vi "Main_ver4.vi"(0 "PID On":bool) -> (5 "Total (V)":dbl[](array[slide]) scale=-8.0..8.0, 6 "Force (N)":T1(graph)={"M1 ref force"=19.748953974895397, "M2 ref force"=19.748953974895397, "M1 mes force"=8.73009296352717, "M2 mes force"=8.373055442726807})   [LabVIEW 2021]
uses:
  <vilib>/addons/control/pid/NI_PID_pid.lvlib
  <vilib>/platform/TimedLoop/XDataNode/XDataNode.xnode
  <vilib>/Platform/TimedLoop/XDataNode/nitl_modes.ctl
  <vilib>/Platform/TimedLoop/XDataNode/XDNodeRunTimeDep.lvlib
  <vilib>/Platform/TimedLoop/XDataNode/wakeup.ctl
  <vilib>/Platform/TimedLoop/XDataNode/timing_clust.ctl
  <vilib>/Analysis/NI_AALBase.lvlib
  <vilib>/DAQmx/configure/timing.llb/DAQmx Timing (Sample Clock).vi
  <vilib>/ptbypt/NI_PtbyPt.lvlib
  <vilib>/Analysis/3filter.llb/Filter Passband Type.ctl
  <vilib>/DAQmx/create/channels.llb/DAQmx Create Channel (AI-Voltage-Basic).vi
  <vilib>/DAQmx/create/channels.llb/DAQmx Create Channel (DO-Digital Output).vi
  <vilib>/addons/control/pid/pid.llb/PID (DBL).vi
  <vilib>/DAQmx/write.llb/DAQmx Write (Digital 1D Bool 1Chan 1Samp).vi
  <vilib>/Analysis/baseanly.llb/Real Dot Product.vi
  <vilib>/DAQmx/write.llb/DAQmx Write (Analog 1D DBL NChan 1Samp).vi
  <vilib>/DAQmx/create/channels.llb/DAQmx Create Channel (AO-Voltage-Basic).vi
panel:
  in  "Tab":enum32{"Page 1", "Page 2"}(tab)
  out "RBF Output":dbl(slide)=-2.8000715957430593 scale=-40.0..50.0
  out "Speed":dbl[](array[numeric])=[1.7549382010467513e-60, 1.807415273169756e-52]
  out "Mes Tension":dbl[](array[numeric])=[10.779007592916166, 8.389554321602144]
  out "Mes Position (mm)":dbl[](array[numeric])=[75.36000199819, -48.33317799163001]
  out "Ref Position (mm)":dbl
  out "Ref Tension":dbl[](array[numeric])=[19.748953974895397, 19.748953974895397]
  in  "Tab Control 4":enum32{"GRAPH", "DEVEL"}(tab)
  out "XY Graph":cluster{dbl[], dbl[]}[](graph)=[{[0.0, 26.31578947368421, 52.63157894736842, 78.94736842105263, 105.26315789473684, 131.57894736842104, 157.89473684210526, 184.21052631578945, 210.52631578947367, 236.8421052631579, 263.1578947368421, 289.4736842105263, 315.7894736842105, 342.10526315789474, 368.4210526315789, 394.7368421052631, 421.05263157894734, 447.36842105263156, 473.6842105263158, 499.99999999999994], [-1.87, -1.8414422208867078, -1.7583590718201578, -1.6281335147614857, -1.4618588659589593, -1.2727815045556152, -1.0745713204427367, -0.879730430835235, -0.6983883150844216, -0.5376223240442685, -0.40131981493157487, -0.2904938166741144, -0.20389950050143207, -0.13878048824938563, -0.09159539506910583, -0.058620814615532306, -0.03638002877625406, -0.02189309729851222, -0.012775689731560116, -0.007229270660814157]}, {[0.0, 26.31578947368421, 52.63157894736842, 78.94736842105263, 105.26315789473684, 131.57894736842104, 157.89473684210526, 184.21052631578945, 210.52631578947367, 236.8421052631579, 263.1578947368421, 289.4736842105263, 315.7894736842105, 342.10526315789474, 368.4210526315789, 394.7368421052631, 421.05263157894734, 447.36842105263156, 473.6842105263158, 499.99999999999994], [-0.5809906464511002, -0.7664296918795039, -0.9804116917090333, -1.2161233359855126, -1.462782454638376, -1.706140698730468, -1.9296694582665639, -2.116332899482121, -2.2507021378374863, -2.3210529255377237, -2.3210529255377237, -2.2507021378374863, -2.1163328994821216, -1.9296694582665639, -1.7061406987304686, -1.4627824546383765, -1.2161233359855128, -0.9804116917090334, -0.7664296918795039, -0.5809906464511005]}, {[0.0, 26.31578947368421, 52.63157894736842, 78.94736842105263, 105.26315789473684, 131.57894736842104, 157.89473684210526, 184.21052631578945, 210.52631578947367, 236.8421052631579, 263.1578947368421, 289.4736842105263, 315.7894736842105, 342.10526315789474, 368.4210526315789, 394.7368421052631, 421.05263157894734, 447.36842105263156, 473.6842105263158, 499.99999999999994], [0.006649382639893229, 0.011750901785178288, 0.020136966499166315, 0.03346184464981654, 0.05391861023460723, 0.08424817086570154, 0.12764836352349906, 0.18754392559490007, 0.2671921736253885, 0.3691283859263683, 0.49449753869312374, 0.6423678620027834, 0.8091638187361518, 0.9883757599794155, 1.1706867314629184, 1.3445974595986148, 1.4975345697271418, 1.6173142264869897, 1.6937329518316242, 1.72]}, {[0.0, 26.31578947368421, 52.63157894736842, 78.94736842105263, 105.26315789473684, 131.57894736842104, 157.89473684210526, 184.21052631578945, 210.52631578947367, 236.8421052631579, 263.1578947368421, 289.4736842105263, 315.7894736842105, 342.10526315789474, 368.4210526315789, 394.7368421052631, 421.05263157894734, 447.36842105263156, 473.6842105263158, 499.99999999999994], [-2.444341263811207, -2.5961210109810335, -2.7186337970300247, -2.8107950060971816, -2.8707227103627284, -2.8946740324203812, -2.8765924151858018, -2.808519404722456, -2.6818982792965196, -2.489546863655624, -2.2278752017761745, -1.898828092508817, -1.5110685812474018, -1.080074186536534, -0.627049362336656, -0.17680580965529402, 0.2450312049653749, 0.6150094374794441, 0.9145275702205602, 1.1317800828880853]}]
  in  "RBF":cluster{"STD":dbl, "Number":i32}={"STD"=150.0, "Number"=3}
  out "Weights":dbl[](array[slide])=[-1.87, -2.33, 1.72] scale=0.0..100.0
  in  "State x":cluster{"Number":i32, "x_0":dbl, "x_f":dbl}={"Number"=20, "x_0"=0.0, "x_f"=500.0}
  in  "Initialize":bool
  in  "Init Loadcell":bool
  out "Period":i64=2
  out "Finished Late? [i-1]":bool
  in  "Set Tension":dbl
  in  "Record?":bool
  in  "Trajectory":i32(knob) scale=0.0..2.0
  in  "Tab Control":enum32{"FORCE", "EE POS", "SPEED"}(tab)=enum."EE POS"
  out "Position (mm)":cluster{"Position":dbl, "Output (mm)":dbl}(graph)={"Position"=75.36000199819, "Output (mm)"=0.0}
  out "RPM":cluster{"Filtered x":dbl, "Filtered x":dbl}(graph)={"Filtered x"=1.7549382010467513e-60, "Filtered x"=1.807415273169756e-52}
  in  "RBF":bool=TRUE
  in  "Set Point":dbl(slide)=19.748953974895397 scale=0.0..40.0
  in  "stop":bool
  in  "Tab Control 3":enum32{"SPEED", "ENABLE", "POSITION"}(tab)
  in  "Gains":T2(array[cluster])=[{"proportional gain (Kc)"=0.03, "integral time (Ti, min)"=0.0, "derivative time (Td, min)"=0.0}, {"proportional gain (Kc)"=0.03, "integral time (Ti, min)"=0.0, "derivative time (Td, min)"=0.0}] {"derivative time (Td, min)" format="%.3f"; "integral time (Ti, min)" format="%.3f"; "proportional gain (Kc)" format="%.3f"}
  in  "Damping":dbl[](array[numeric])=[0.002, 0.002]
  out "Output (V)":dbl[](array[slide])=[3.509876402093503e-63, 3.614830546339512e-55] scale=-8.0..10.0
  in  "Motor Enable":bool[](array[boolean])=[FALSE, FALSE]
  in  "PID gains":T3={"proportional gain (Kc)"=0.1, "integral time (Ti, min)"=0.0, "derivative time (Td, min)"=0.0} {"derivative time (Td, min)" format="%.3f"; "integral time (Ti, min)" format="%.3f"; "proportional gain (Kc)" format="%.3f"}
  out "Ref Tension Output":dbl(slide)=-7.536000199819 scale=-40.0..40.0
  in  "Position PID On":bool
  # "MONITOR"
  # "ADAPTIVE LEARNING"
  # "TUNE"
  # "CONTROL"
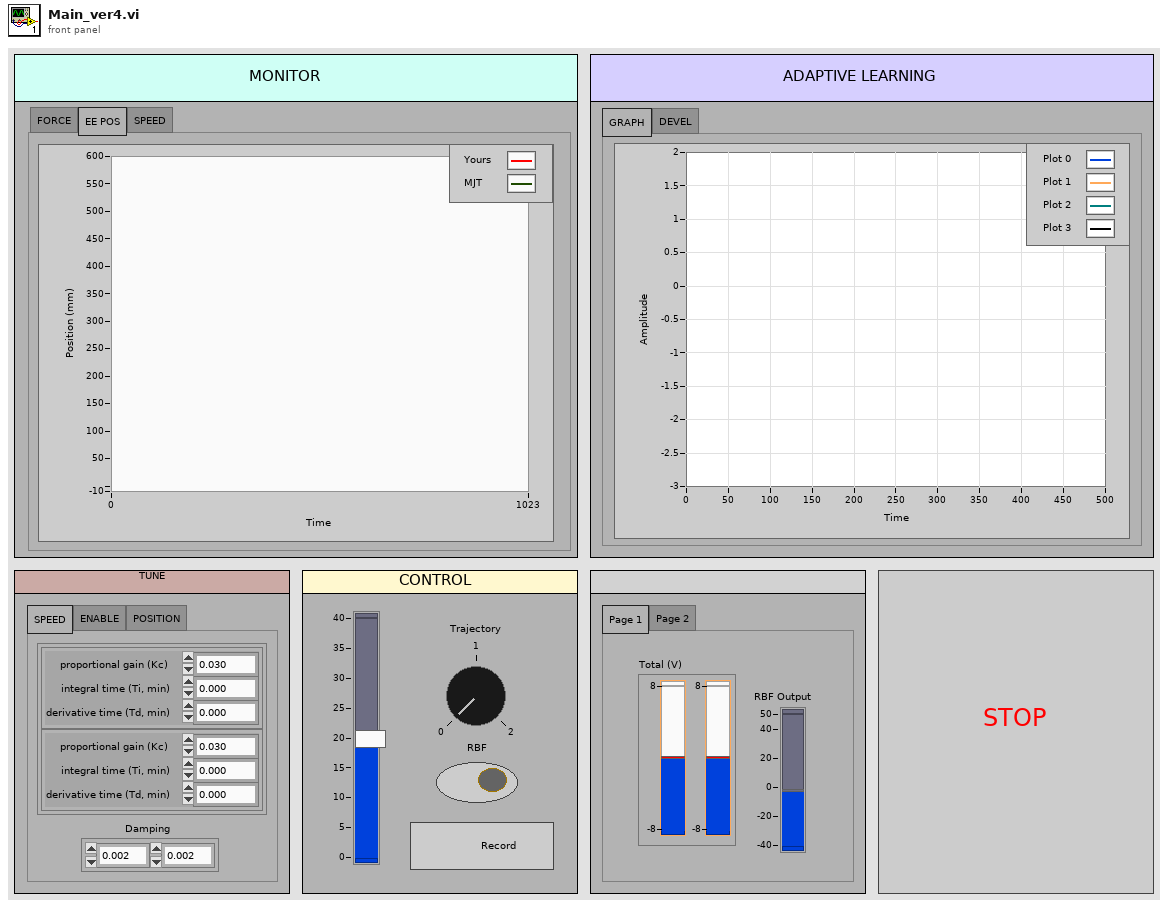
[diagram p1: front panel]
types:
  T1 = cluster{"M1 ref force":dbl, "M2 ref force":dbl, "M1 mes force":dbl, "M2 mes force":dbl}
  T2 = cluster{"proportional gain (Kc)":dbl, "integral time (Ti, min)":dbl, "derivative time (Td, min)":dbl}[]
  T3 = cluster{"proportional gain (Kc)":dbl, "integral time (Ti, min)":dbl, "derivative time (Td, min)":dbl}
  T4 = enum16{"open", "open or create", "create or replace", "create", "open (read-only)"}
  T5 = typedef "XDNodeRunTimeDep.lvlib/timing_clust.ctl" = cluster{"Expected End [f-1]":u64, "Actual End [f-1]":u64, "Finished Late? [f-1]":bool, "Expected End [i-1]":u64, "Actual End [i-1]":u64, "Finished Late? [i-1]":bool, "Expected Start [i]":u64, "Actual Start [i]":u64, "Expected Start [f]":u64, "Actual Start [f]":u64, "Source Name":string, "Structure Name":string, "Period":i64, "Deadline":i64, "Offset":i64, "Start":i64, "Priority":i32, "Timeout":i32, "Mode":T6, "Wakeup Reason":T7, "Error":errorcluster, "Source Type":string, "Secondary Source Type":string, "Global End Time":u64, "Global Start Time":u64, "Frame Duration":u64, "Iteration Duration":u64, "Assigned CPU":i32, "I/O Scan Engine Mode":u32}
  T6 = typedef "XDNodeRunTimeDep.lvlib/nitl_modes.ctl" = enum32{"No Change", "Process missed periods, maintain original phase", "Discard missed periods, maintain original phase", "Process missed periods, ignore original phase", "Discard missed periods, ignore original phase"}
  T7 = typedef "XDNodeRunTimeDep.lvlib/wakeup.ctl" = enum32{"Normal", "Aborted", "Asynchronous wakeup", "Timing source error", "Timed loop error", "Timeout"}
  T8 = typedef "NI_AALBase.lvlib/Filter Passband Type.ctl" = enum32{"Lowpass", "Highpass", "Bandpass", "Bandstop"}
  T9 = cluster{"Set Point":dbl, "Set Point":dbl, "Filtered x":dbl, "Filtered x":dbl}
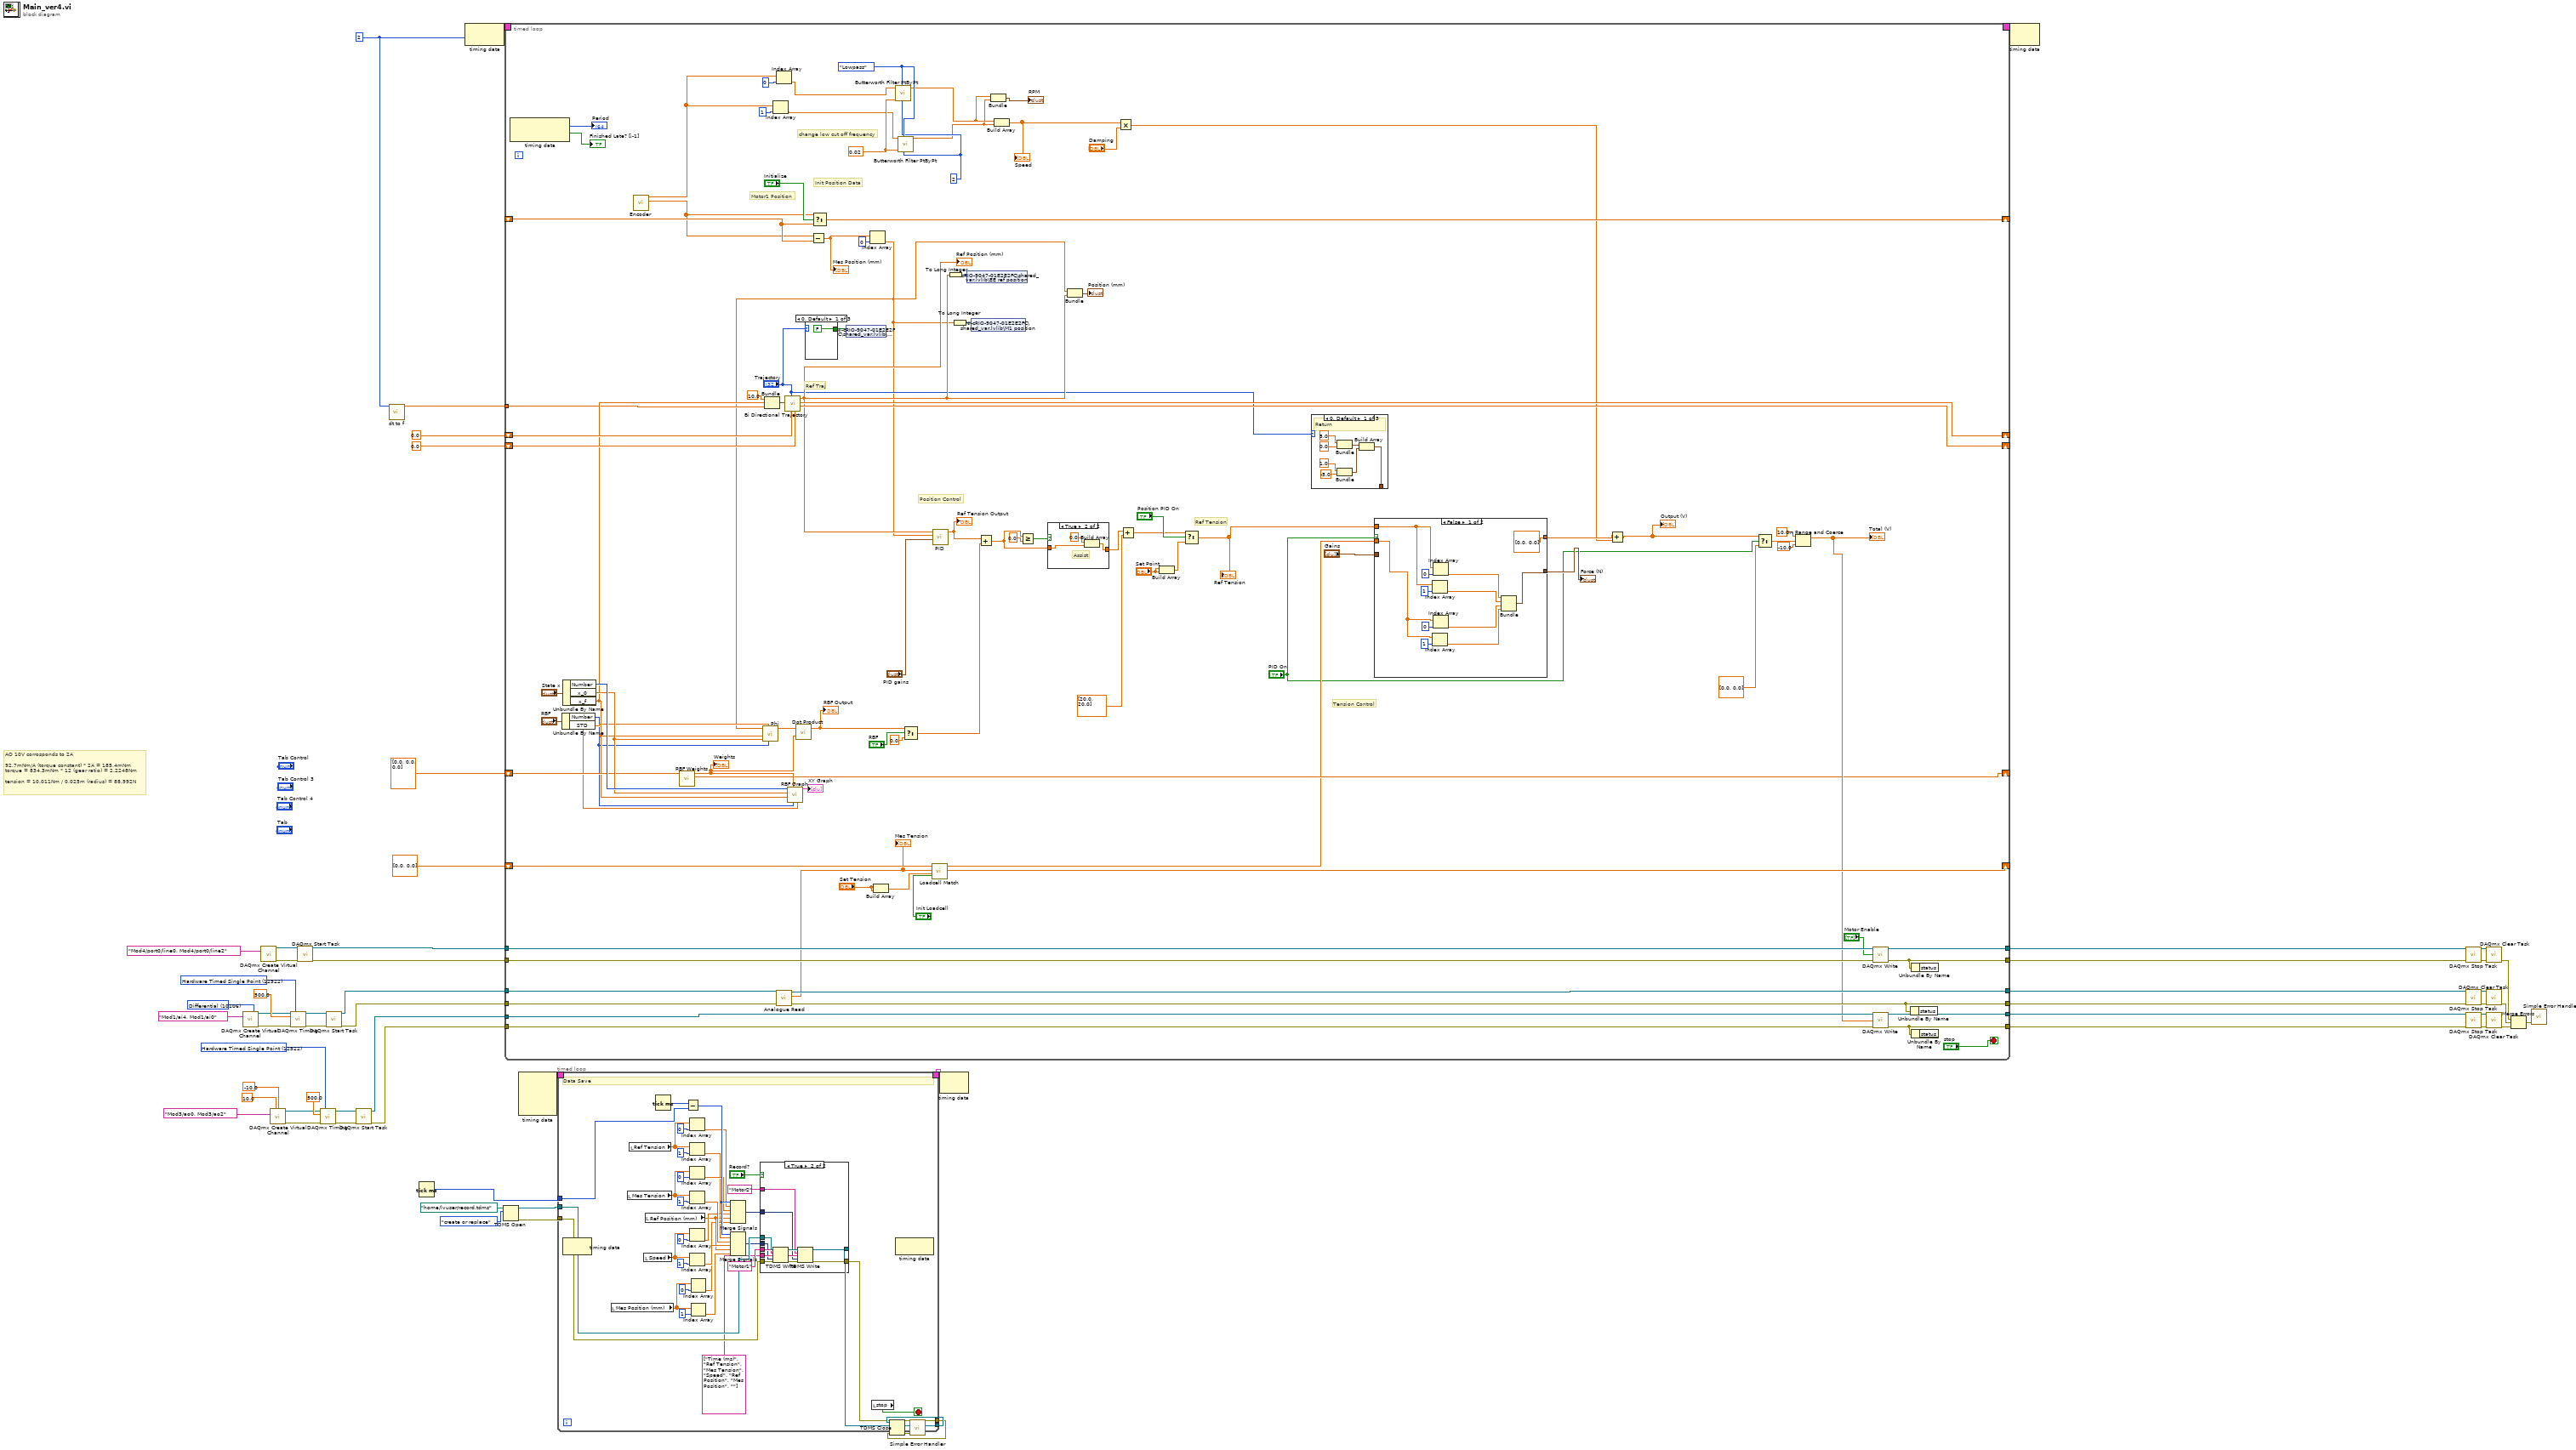
[diagram p0: block diagram]
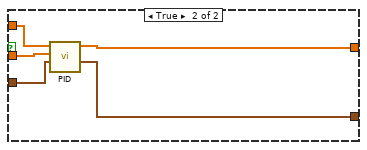
[diagram p3: hidden frame]
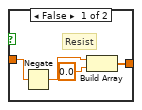
[diagram p4: hidden frame]
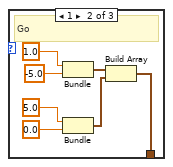
[diagram p5: hidden frame]
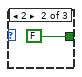
[diagram p7: hidden frame]
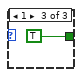
[diagram p8: hidden frame]
diagram:
  w16 = 12522 items=["Finite Samples"=10178, "Continuous Samples"=10123, "Hardware Timed Single Point"=12522] ("sample mode")
  w19 = 12522 items=["Finite Samples"=10178, "Continuous Samples"=10123, "Hardware Timed Single Point"=12522] ("sample mode")
  w26 = i64 2 ("Period")
  w32 = 10106 items=["Default"=-1, "RSE"=10083, "NRSE"=10078, "Differential"=10106, "Pseudodifferential"=12529] ("input terminal configuration")
  # "AO 10V corrosponds to 2A\n\n92.7mNm/A (torque constant) * 2A = 185.4mNm\ntorque = 834.3mNm * 12 (gear ratio) = 2.2248Nm\n\ntension = 10.011Nm / 0.025m (radius) = 88.992N"
  n1 = call-poly <vilib>:"DAQmx Create Virtual Channel.vi"("input terminal configuration"=w32, "physical channels"=tag "Mod1/ai4, Mod1/ai0") -> ("task out"=w23:refnum<k21>, "error out"=w22:errorcluster)  [unwired: 12 in]
  n2 = call-poly <vilib>:"DAQmx Create Virtual Channel.vi"("lines"=tag "Mod4/port0/line0, Mod4/port0/line2") -> ("task out"=w18:refnum<k21>, "error out"=w54:errorcluster)  [unwired: 13 in]
  n3 = call-poly <vilib>:"DAQmx Create Virtual Channel.vi"("maximum value"=10.0 ("AO max"), "minimum value"=-10.0 ("AO min"), "physical channels"=tag "Mod3/ao0, Mod3/ao2" ("Physical Channel(s)")) -> ("task out"=w15:refnum<k21>, "error out"=w13:errorcluster)  [unwired: 11 in]
  n4 = call-poly <vilib>:"DAQmx Timing.vi"("task/channels in"=w23, "sample mode"=w19, "rate"=500.0, "error in"=w22) -> ("task out"=w20:refnum<k21>, "error out"=w21:errorcluster)  [unwired: 10 in]
  n5 = call <vilib>:"DAQmx Start Task.vi"("task/channels in"=w18, "error in"=w54) -> ("task out"=w52:refnum<k21>, "error out"=w51:errorcluster)  [unwired: 12 in]
  n6 = call-poly <vilib>:"DAQmx Timing.vi"("task/channels in"=w15, "sample mode"=w16, "rate"=500.0, "error in"=w13) -> ("task out"=w14:refnum<k21>, "error out"=w12:errorcluster)  [unwired: 10 in]
  n7 = call <vilib>:"DAQmx Start Task.vi"("task/channels in"=w20, "error in"=w21) -> ("task out"=w45:refnum<k21>, "error out"=w44:errorcluster)  [unwired: 12 in]
  n8 = call <vilib>:"DAQmx Start Task.vi"("task/channels in"=w14, "error in"=w12) -> ("task out"=w56:refnum<k21>, "error out"=w55:errorcluster)  [unwired: 12 in]
  n9 = call "dt to f.vi"("Period"=w26) -> ("Frequency"=w25:dbl)  [unwired: 10 in]
  n10 = Tick Count (ms)() -> (millisecond timer value=w4:u32)
  n11 = node-c288(w26) -> (w28:T5)
  n12 = TDMS Open(10:T4."create or replace" ("operation (0:open)"), 11:path "/home/lvuser/record.tdms" ("file path")) -> (0:w7:errorcluster, 3:w11:refnum<k34>)  [unwired: 5 in]
  n13 = timed-loop {
    tunnel: [w155] -> w60
    tunnel: [w154] -> w59
    tunnel: [w141] -> w58
    tunnel: [w146] -> w57
    tunnel: w45 -> [w152]
    tunnel: w44 -> [w151]
    tunnel: w56 -> [w140]
    tunnel: w55 -> [w153]
    tunnel: w52 -> [w150]
    tunnel: w51 -> [w149]
    tunnel: [w148] -> w48
    tunnel: [w147] -> w47
    shift-right: [w144] -> _
    shift-left: 0.0 ("total time") -> [w145]
    shift-right: [w143] -> _
    shift-left: _ -> [w142]
    shift-right: [w138] -> _
    shift-left: dbl[] [0.0, 0.0] ("measured force") -> [w139]
    shift-right: [w136] -> _
    shift-left: 0.0 ("total time") -> [w137]
    timing: w28 -> [_]
    timing-out: [_] -> w27
    shift-right: [w106] -> _
    shift-left: dbl[] [0.0, 0.0, 0.0] ("Array of Double") -> [w107]
    tunnel: w25 -> [w98]
    stop <- "stop" stop-if-true
    w89 = 2 ("order")
    w91 = 0.02 ("low cutoff freq: fl")
    w90 = Filter_Passband_Type."Lowpass" ("filter type")
    # "Tension Control"
    # "change low cut off frequency"
    # "Ref Tension"
    # "Position Control"
    # "Ref Traj"
    # "Init Position Data"
    # "Motor1 Position"
    n14 = node-c288() -> (→"Period":i64, →"Finished Late? [i-1]":bool)  [unwired: 1 in]
    n15 = Unbundle By Name("RBF") -> ("Number"=w94:i32, "STD"=w95:dbl)
    n16 = Unbundle By Name("State x") -> ("Number"=w116:i32, "x_0"=w113:dbl, "x_f"=w99:dbl)
    n17 = call "Encoder.vi"() -> ("Mes Pos (mm)"=w78:dbl[], "RPM"=w86:dbl[])  [unwired: 10 in]
    n18 = call "RBF Weights.vi"("Array of Double in"=w107) -> ("Array of Double out"=w106:dbl[], "Array of Double 3"=w108:dbl[])  [unwired: 9 in]
    "Weights" <- w108
    n19 = Bundle("y"=10.0, "x_f"=w99, "Frequency"=w98) -> (w97:cluster{"y":dbl, "x_f":dbl, "Frequency":dbl})  [unwired: 1 in]
    n20 = Index Array(array=w86, index=1) -> (element=w84:dbl)
    n21 = Index Array(array=w86, index=0) -> (element=w85:dbl)
    n22 = call "Analogue Read.vi"("error in"=w151, "task/channels in"=w152) -> ("error out"=w146:errorcluster, "measured force"=w123:dbl[], "task out"=w141:refnum<k21>)  [unwired: 6 in, 1 out]
    "Mes Tension" <- w123
    n23 = call "Bi Directional Trajectory.vi"("Return Time"=w137, "Go Time"=w145, "Traj Start"="Trajectory", "Trajectory Settings"=w97) -> ("Return Next Time"=w136:dbl, "Go Next Time"=w144:dbl, "Output (mm)"=w112:dbl)  [unwired: 5 in]
    "Ref Position (mm)" <- w112
    n24 = call "RBF Graph.vi"("STD"=w95, "Number"=w94, "Array of Double 3"=w108, "x_f"=w99, "x_0"=w113, "Number 2"=w116) -> ("Array"=→"XY Graph":cluster{dbl[], dbl[]}[])  [unwired: 5 in]
    n25 = case shown="0, Default" "Trajectory" {
      tunnel: [FALSE FALSE TRUE] -> w109
      frame 0, Default {
      }
      frame 2 {
      }
      frame 1 {
      }
    }
    n26 = Subtract(x=w78, y=w142) -> (x-y=w77:dbl[])
    "Mes Position (mm)" <- w77
    n27 = Select(t=w78, s="Initialize", f=w142) -> (s? t:f=w143:dbl[])
    n28 = shared-variable "NI-cRIO-9047-01E2E2FC\\shared_var.lvlib\\Trigger"(w109) -> ()  [unwired: 1 in, 1 out]
    n29 = Index Array(array=w77, index=0) -> (element=w63:dbl)
    n30 = call "Phi.vi"("Number"=w94, "STD"=w95, "x_f"=w99, "x_0"=w113, "Output (mm)"=w63) -> ("Array"=w111:dbl[])  [unwired: 6 in]
    n31 = call-poly <vilib>:"Dot Product.vi"("Y Vector"=w108, "X Vector"=w111) -> ("X * Y"=w105:dbl)  [unwired: 1 out]
    "RBF Output" <- w105
    n32 = Build Array("Set Tension", "Set Tension") -> (w61:dbl[])
    n33 = call <vilib>:"Butterworth Filter PtByPt.vi"("order"=w89, "filter type"=w90, "low cutoff freq: fl"=w91, "x"=w85) -> ("Filtered x"=w75:dbl)  [unwired: 5 in, 1 out]
    n34 = call <vilib>:"Butterworth Filter PtByPt.vi"("order"=w89, "filter type"=w90, "low cutoff freq: fl"=w91, "x"=w84) -> ("Filtered x"=w74:dbl)  [unwired: 5 in, 1 out]
    n35 = Select(t=w105, s="RBF", f=0.0) -> (s? t:f=w64:dbl)
    n36 = call "Loadcell Match.vi"("Initialize"="Init Loadcell", "Set Tension"=w61, "Mes Tension"=w123, "Next Tension Error"=w139) -> ("Tension Error"=w138:dbl[], "Filtered Tension"=w71:dbl[])  [unwired: 6 in]
    n37 = call-poly <vilib>:"PID.vi"("PID gains"="PID gains", "process variable"=w63, "setpoint"=w112) -> ("output"=w66:dbl)  [unwired: 7 in, 1 out]
    "Ref Tension Output" <- w66
    n38 = To Long Integer(number=w112) -> (32bit integer=w120:i32)
    n39 = To Long Integer(number=w63) -> (32bit integer=w119:i32)
    n40 = shared-variable "NI-cRIO-9047-01E2E2FC\\shared_var.lvlib\\EE ref position"(w120) -> ()  [unwired: 1 in, 1 out]
    n41 = shared-variable "NI-cRIO-9047-01E2E2FC\\shared_var.lvlib\\M1 position"(w119) -> ()  [unwired: 1 in, 1 out]
    n42 = Add(x=w66, y=w64) -> (x+y=w65:dbl)
    n43 = Bundle("Filtered x"=w75, "Filtered x"=w74) -> (→"RPM":cluster{"Filtered x":dbl, "Filtered x":dbl})  [unwired: 1 in]
    n44 = Build Array(w75, w74) -> (w72:dbl[])
    "Speed" <- w72
    n45 = Greater Or Equal?(x=w65, y=0.0) -> (x >= y?=w104:bool)
    n46 = case shown="True" w104 {
      tunnel: w65 -> [w177 w180]
      tunnel: [w179 w182] -> w101
      frame False {
        # "Resist"
        n47 = Negate(x=w177) -> (-x=w176:dbl)
        n48 = Build Array(w176, 0.0 ("element")) -> (w179:dbl[])
      }
      frame True {
        # "Assist"
        n49 = Build Array(0.0 ("element"), w180) -> (w182:dbl[])
      }
    }
    n50 = Bundle("Position"=w63, "Output (mm)"=w112) -> (→"Position (mm)":cluster{"Position":dbl, "Output (mm)":dbl})  [unwired: 1 in]
    n51 = Multiply(x=w72, y="Damping") -> (x*y=w76:dbl[])
    n52 = Add(x=w101, y=dbl[] [20.0, 20.0] ("x")) -> (x+y=w100:dbl[])
    n53 = Build Array("Set Point", "Set Point") -> (w131:dbl[])
    n54 = Select(t=w100, s="Position PID On", f=w131) -> (s? t:f=w67:dbl[])
    "Ref Tension" <- w67
    n55 = case shown="0, Default" "Trajectory" {
      tunnel: [w183 w190 _] -> _
      frame 0, Default {
        # "Return"
        n56 = Bundle(5.0, 0.0) -> (w189:cluster{dbl, dbl})  [unwired: 1 in]
        n57 = Bundle(1.0, -5.0) -> (w188:cluster{dbl, dbl})  [unwired: 1 in]
        n58 = Build Array(w189, w188) -> (w183:cluster{dbl, dbl}[])
      }
      frame 1 {
        # "Go"
        n59 = Bundle(1.0, -5.0) -> (w191:cluster{dbl, dbl})  [unwired: 1 in]
        n60 = Bundle(5.0, 0.0) -> (w192:cluster{dbl, dbl})  [unwired: 1 in]
        n61 = Build Array(w191, w192) -> (w190:cluster{dbl, dbl}[])
      }
      frame 2 {
      }
    }
    n62 = case shown="False" "PID On" {
      tunnel: [dbl[] [0.0, 0.0] ("PID output") w172] -> w82
      tunnel: w71 -> [w159 w171]
      tunnel: "Gains" -> [_ w170]
      tunnel: [w158 w169] -> w69
      tunnel: w67 -> [w157 w168]
      frame False {
        n63 = Index Array(array=w157, index=1) -> (element=w162:dbl)
        n64 = Index Array(array=w159, index=1) -> (element=w160:dbl)
        n65 = Index Array(array=w157, index=0) -> (element=w163:dbl)
        n66 = Index Array(array=w159, index=0) -> (element=w161:dbl)
        n67 = Bundle("Set Point"=w163, "Set Point"=w162, "Filtered x"=w161, "Filtered x"=w160) -> (w158:T9)  [unwired: 1 in]
      }
      frame True {
        n68 = call <vilib>:"PID.vi"("PID gains"=w170, "mes force"=w171, "ref force"=w168) -> ("output cluster"=w169:T1, "PID output"=w172:dbl[])  [unwired: 7 in]
      }
    }
    "Force (N)" <- w69
    n69 = Add(x=w82, y=w76) -> (x+y=w81:dbl[])
    "Output (V)" <- w81
    n70 = Select(t=w81, s="PID On", f=dbl[] [0.0, 0.0]) -> (s? t:f=w133:dbl[])
    n71 = In Range and Coerce(upper limit=10.0, x=w133, lower limit=-10.0) -> (coerced(x)=w121:dbl[])  [unwired: 1 out]
    "Total (V)" <- w121
    n72 = call-poly <vilib>:"DAQmx Write.vi"("task/channels in"=w150, "data"="Motor Enable", "error in"=w149) -> ("task out"=w148:refnum<k21>, "error out"=w147:errorcluster)  [unwired: 10 in, 1 out]
    n73 = call-poly <vilib>:"DAQmx Write.vi"("task/channels in"=w140, "data"=w121, "error in"=w153) -> ("task out"=w155:refnum<k21>, "error out"=w154:errorcluster)  [unwired: 10 in, 1 out]
    n74 = Unbundle By Name(w146) -> ()  [unwired: 1 out]
    n75 = Unbundle By Name(w147) -> ()  [unwired: 1 out]
    n76 = Unbundle By Name(w154) -> ()  [unwired: 1 out]
  }
  n77 = node-c288() -> (w3:T5)  [unwired: 4 in]
  n78 = timed-loop {
    tunnel: w11 -> [w235]
    tunnel: [w224] -> w10
    tunnel: [w232] -> w8
    tunnel: w7 -> [w234]
    tunnel: w4 -> [w226]
    timing: w3 -> [_]
    timing-out: [_] -> w2
    stop <- w222 stop-if-true
    # "Data Save"
    n79 = node-c288() -> ()  [unwired: 1 in, 1 out]
    n80 = local read "Mes Position (mm)"() -> (w208:dbl[])
    n81 = local read "Mes Tension"() -> (w219:dbl[])
    n82 = local read "Ref Tension"() -> (w203:dbl[])
    n83 = local read "Speed"() -> (w214:dbl[])
    n84 = local read "Ref Position (mm)"() -> (w209:dbl)
    n85 = Tick Count (ms)() -> (millisecond timer value=w227:u32)
    n86 = Subtract(x=w227, y=w226) -> (x-y=w225:u32)
    n87 = Index Array(array=w203, index=0) -> (element=w202:dbl)
    n88 = Index Array(array=w203, index=1) -> (element=w201:dbl)
    n89 = Index Array(array=w219, index=0) -> (element=w218:dbl)
    n90 = Index Array(array=w219, index=1) -> (element=w217:dbl)
    n91 = Index Array(array=w214, index=0) -> (element=w212:dbl)
    n92 = Index Array(array=w214, index=1) -> (element=w213:dbl)
    n93 = Index Array(array=w208, index=0) -> (element=w207:dbl)
    n94 = Index Array(array=w208, index=1) -> (element=w206:dbl)
    n95 = Merge Signals(w225, w202, w218, w212, w209, w207) -> (w228:dynamicdata)
    n96 = Merge Signals(w225, w201, w217, w213, w209, w206) -> (w229:dynamicdata)
    n97 = case shown="True" "Record?" {
      tunnel: w235 -> [w236 w249]
      tunnel: w234 -> [w237 w248]
      tunnel: "Motor1" ("group name in (Untitled)") -> [_ w247]
      tunnel: [w237 w245] -> w232
      tunnel: [w236 w243] -> w224
      tunnel: "Motor2" ("group name in (Untitled)") -> [_ w242]
      tunnel: string[] ["Time (ms)", "Ref Tension", "Mes Tension", "Speed", "Ref Position", "Mes Position", ""] ("channel name(s) in (Untitled)") -> [_ w241]
      tunnel: w229 -> [_ w239]
      tunnel: w228 -> [_ w238]
      frame False {
      }
      frame True {
        n98 = TDMS Write(0:w249, 5:w247, 7:w241, 9:w239, 11:w248) -> (4:w244:refnum<k34>, 8:w240:string[], 15:w246:errorcluster)  [unwired: 1 in, 1 out]
        n99 = TDMS Write(0:w244, 5:w242, 7:w240, 9:w238, 11:w246) -> (4:w243:refnum<k34>, 15:w245:errorcluster)  [unwired: 1 in, 2 out]
      }
    }
    n100 = local read "stop"() -> (w222:bool)
    n101 = node-c288() -> ()  [unwired: 1 in, 1 out]
  }
  n102 = TDMS Close(8:w8, 11:w10) -> (0:w9:errorcluster)  [unwired: 1 out]
  n103 = call <vilib>:"Simple Error Handler.vi"("error in (no error)"=w9) -> ()  [unwired: 4 in, 5 out]
  n104 = node-c288(w2) -> ()  [unwired: 1 out]
  n105 = node-c288(w27) -> ()  [unwired: 1 out]
  n106 = call <vilib>:"DAQmx Stop Task.vi"("task/channels in"=w48, "error in"=w47) -> ("task out"=w50:refnum<k21>, "error out"=w49:errorcluster)  [unwired: 12 in]
  n107 = call <vilib>:"DAQmx Stop Task.vi"("task/channels in"=w58, "error in"=w57) -> ("task out"=w38:refnum<k21>, "error out"=w37:errorcluster)  [unwired: 12 in]
  n108 = call <vilib>:"DAQmx Stop Task.vi"("task/channels in"=w60, "error in"=w59) -> ("task out"=w40:refnum<k21>, "error out"=w39:errorcluster)  [unwired: 12 in]
  n109 = call <vilib>:"DAQmx Clear Task.vi"("task in"=w50, "error in"=w49) -> ("error out"=w33:errorcluster)  [unwired: 13 in]
  n110 = call <vilib>:"DAQmx Clear Task.vi"("task in"=w38, "error in"=w37) -> ("error out"=w34:errorcluster)  [unwired: 13 in]
  n111 = call <vilib>:"DAQmx Clear Task.vi"("task in"=w40, "error in"=w39) -> ("error out"=w35:errorcluster)  [unwired: 13 in]
  n112 = Merge Errors(w33, w34, w35) -> (w36:errorcluster)
  n113 = call <vilib>:"Simple Error Handler.vi"("error in (no error)"=w36) -> ()  [unwired: 4 in, 5 out]
